vi "read data.vi"() -> ()   [LabVIEW 2016]
panel:
  out "Waveform Chart":dbl(graph)
  out "data":dbl
  in  "stop":bool
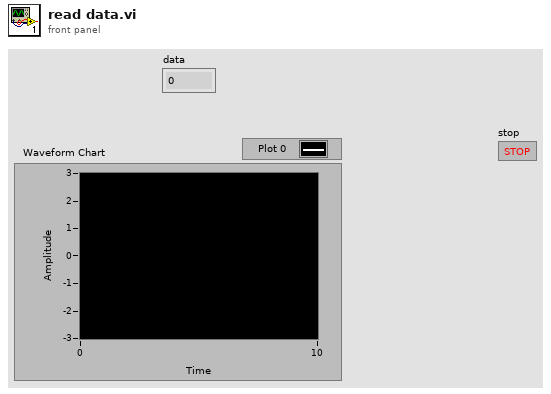
[diagram p1: front panel]
types:
  T1 = enum16{"Read", "Write", "ReadWrite", "BufferedRead", "BufferedReadWrite"}
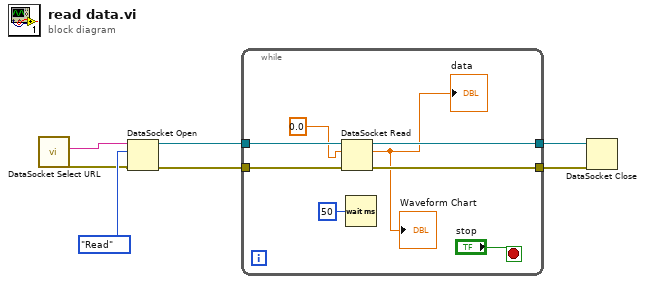
[diagram p0: block diagram]
diagram:
  n1 = call <vilib>:"DataSocket Select URL.vi"() -> ("error out"=w4:errorcluster, "URL"=w7:string)  [unwired: 9 in, 1 out]
  n2 = DataSocket Open(8:w4, 10:T1."Read" ("mode"), 11:w7) -> (0:w5:errorcluster, 3:w3:refnum<k13>)  [unwired: 1 in]
  n3 = while {
    tunnel: w5 -> [w14]
    tunnel: w3 -> [w13]
    tunnel: [w12] -> w2
    tunnel: [w11] -> w1
    stop <- "stop" stop-if-true
    n4 = DataSocket Read(8:w14, 10:0.0, 11:w13) -> (0:w11:errorcluster, 2:→"data" →"Waveform Chart":dbl, 3:w12:refnum<k13>)  [unwired: 2 in, 4 out]
    n5 = Wait (ms)(milliseconds to wait=u32 50) -> ()  [unwired: 1 out]
  }
  n6 = DataSocket Close(8:w1, 11:w2) -> ()  [unwired: 1 in, 2 out]
